vi "kursory.vi"() -> ()   [LabVIEW 2013]
uses:
  <vilib>/Utility/miscctls.llb/LVPointDoubleTypeDef.ctl
  <vilib>/Utility/miscctls.llb/LVCursorListTypeDef.ctl
  Kontrolki/GUI/Wysw_kursorow.ctl
  <vilib>/measure/NI_MABase.lvlib
panel:
  out "Data":T1
  in  "Create meas Cursor":bool
  in  "Delete cursor":bool
  in  "Create cursor":bool
  in  "Color Box":u32(colorbox)
  in  "Cursor List 2":T2
  in  "Free cursor":bool
  in  "stop":bool
  in  "Listbox":i32(listbox)
  out "Cursor List":T2
  out "Cursor.Cursor Position":T3
  out "Waveform Graph":waveform(dbl)[](graph)
  in  "Array":T4(array[cluster])=[{"signal type"=enum."Sine Wave", "frequency"=10.0, "amplitude"=2.0}, {"signal type"=enum."Sine Wave", "frequency"=13.0, "amplitude"=1.0}, {"signal type"=enum."Sine Wave", "frequency"=7.0, "amplitude"=1.0}, {"signal type"=enum."Sine Wave", "frequency"=5.0, "amplitude"=3.0}] {"amplitude" format="%0.2p"; "frequency" format="%0.2p"}
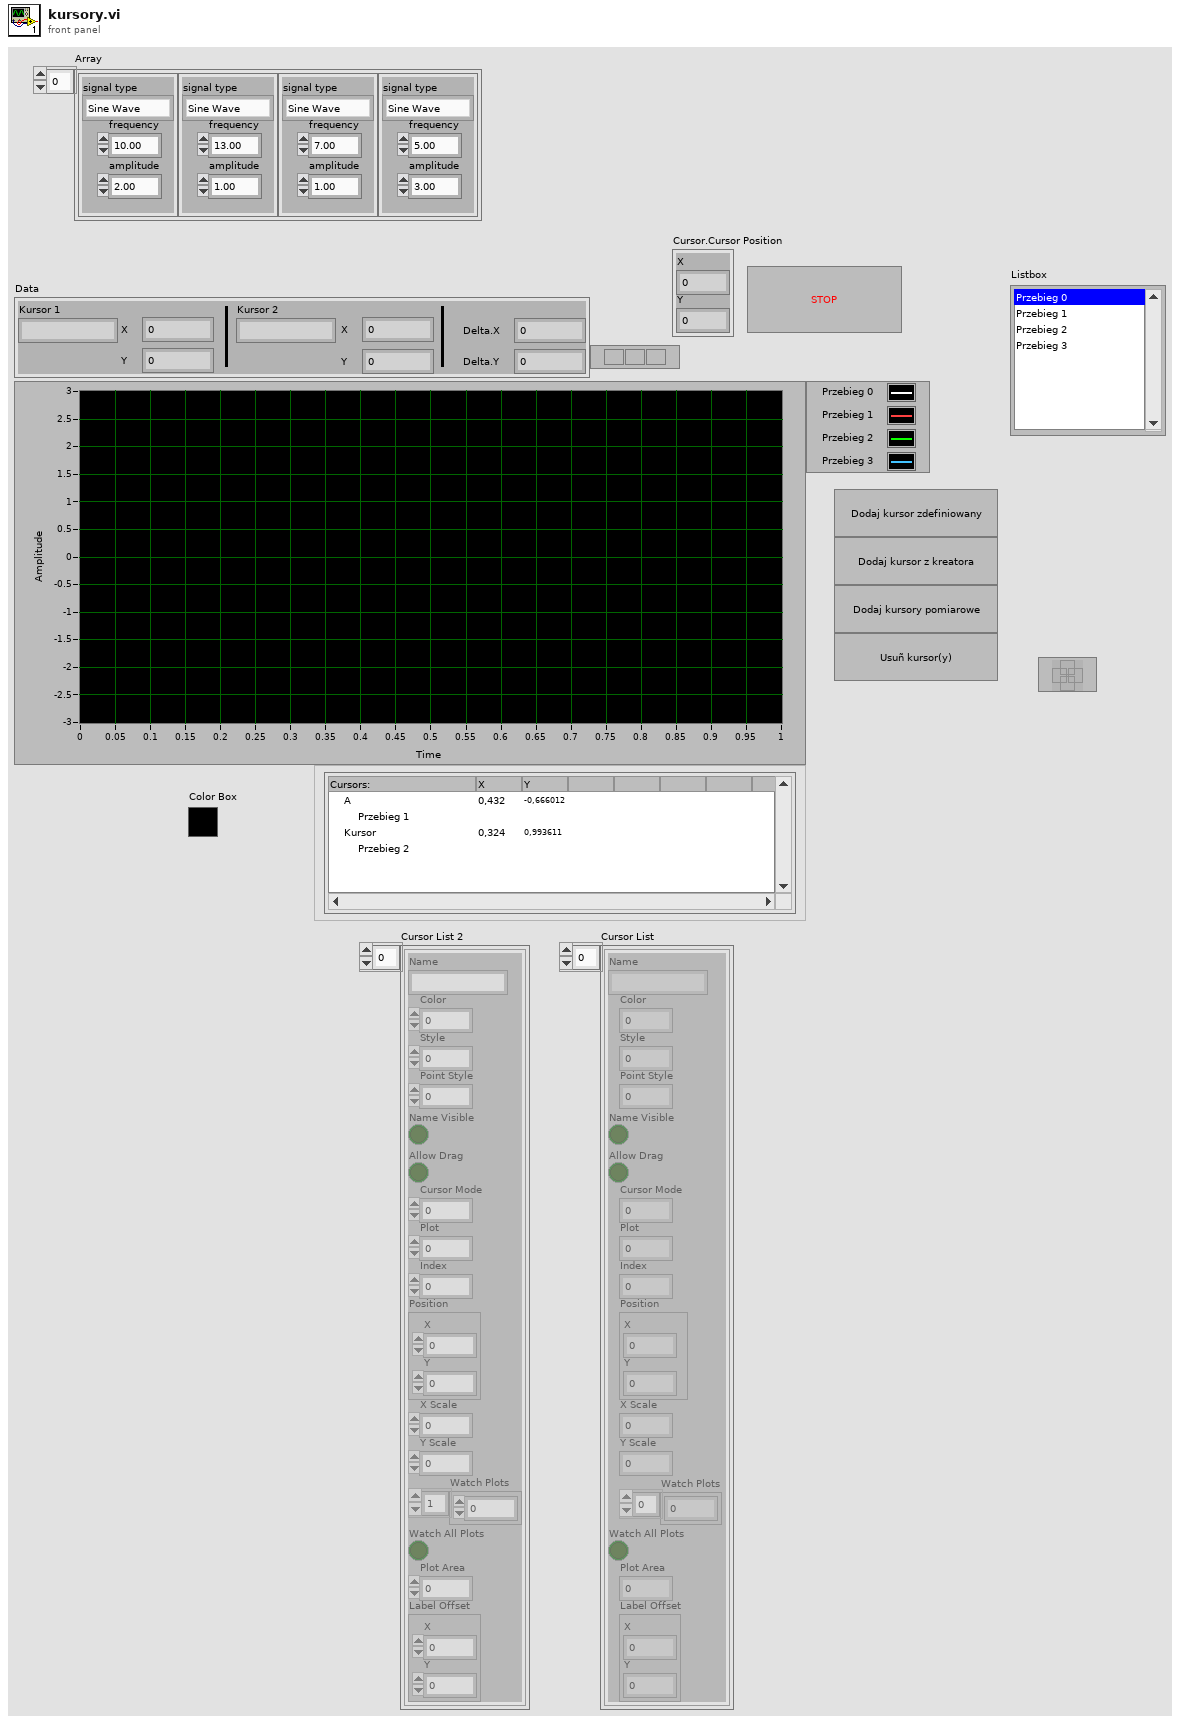
[diagram p1: front panel]
types:
  T1 = typedef "Wysw_kursorow.ctl" = cluster{"Pos.X1":dbl, "Pos.Y1":dbl, "Pos.X2":dbl, "Pos.Y2":dbl, "Delta.X":dbl, "Delta.Y":dbl, "Nazwa.1":string, "Nazwa.2":string}
  T2 = typedef "LVCursorListTypeDef.ctl" = cluster{"Name":string, "Color":u32, "Style":u8, "Point Style":u8, "Name Visible":bool, "Allow Drag":bool, "Cursor Mode":u32, "Plot":i32, "Index":i32, "Position":cluster{"X":dbl, "Y":dbl}, "X Scale":u32, "Y Scale":u32, "Watch Plots":i32[], "Watch All Plots":bool, "Plot Area":i32, "Label Offset":cluster{"X":dbl, "Y":dbl}}[]
  T3 = typedef "LVPointDoubleTypeDef.ctl" = cluster{"X":dbl, "Y":dbl}
  T4 = cluster{"signal type":enum16{"Sine Wave", "Triangle Wave", "Square Wave", "Sawtooth Wave"}, "frequency":dbl, "amplitude":dbl}[]
  T5 = enum16{"Sine Wave", "Triangle Wave", "Square Wave", "Sawtooth Wave"}
  T6 = cluster{"Name":string, "Color":u32, "Style":u8, "Point Style":u8, "Name Visible":bool, "Allow Drag":bool, "Cursor Mode":u32, "Plot":i32, "Index":i32, "Position":cluster{"X":dbl, "Y":dbl}, "X Scale":u32, "Y Scale":u32, "Watch Plots":i32[], "Watch All Plots":bool, "Plot Area":i32, "Label Offset":cluster{"X":dbl, "Y":dbl}}
  T7 = cluster{"Name":string, "Color":u32, "Style":u8, "Point Style":u8, "Name Visible":bool, "Allow Drag":bool, "Cursor Mode":u32, "Plot":i32, "Index":i32, "Position":cluster{"X":dbl, "Y":dbl}, "X Scale":u32, "Y Scale":u32, "Watch Plots":i32[], "Watch All Plots":bool, "Plot Area":i32, "Label Offset":cluster{"X":dbl, "Y":dbl}}[]
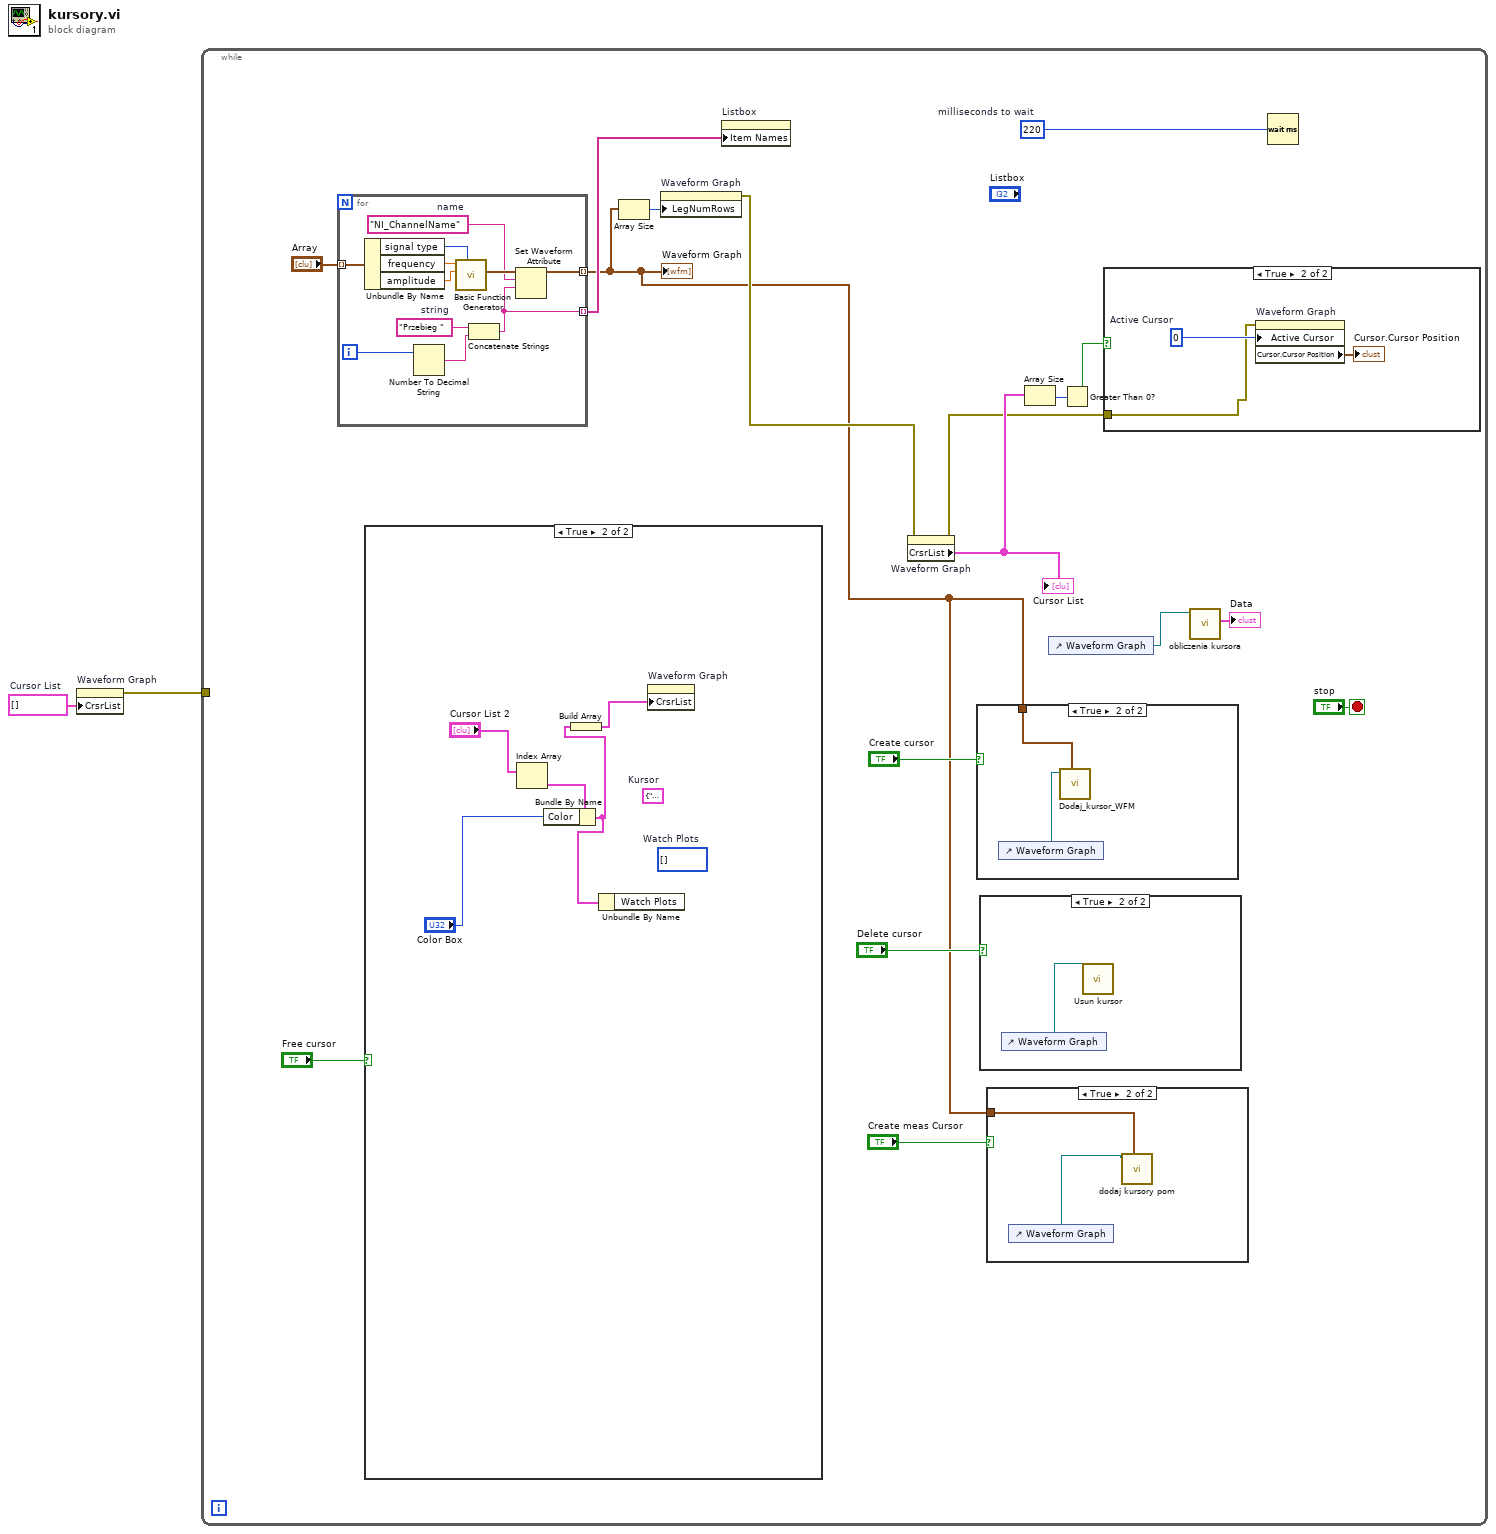
[diagram p0: block diagram]
diagram:
  w2 = T2 []  # Cursor List
  n1 = property on="Waveform Graph" class="WFGraph (strict)"("CrsrList"=w2) -> (error out=w1:errorcluster)  [unwired: 2 in, 1 out]
  n2 = while {
    tunnel: w1 -> [_]
    stop <- "stop" stop-if-true
    w15 = u32 220  # milliseconds to wait
    n3 = for {
      tunnel: "Array" -> [w40] mode=indexing
      tunnel: [w34] -> w4 mode=indexing
      tunnel: [w33] -> w17 mode=indexing
      i -> [w35]
      w37 = "Przebieg "  # string
      w38 = "NI_ChannelName"  # name
      n4 = Unbundle By Name(w40) -> ("signal type"=w43:T5, "frequency"=w42:dbl, "amplitude"=w41:dbl)
      n5 = Number To Decimal String(number=w35) -> (decimal integer string=w36:string)  [unwired: 1 in]
      n6 = call <vilib>:"Basic Function Generator.vi"("signal type"=w43, "amplitude"=w41, "frequency"=w42) -> ("signal out"=w39:waveform(dbl))  [unwired: 6 in, 2 out]
      n7 = Concatenate Strings(w37, w36) -> (w33:string)
      n8 = Set Waveform Attribute(5:w33, 6:w38, 7:w39) -> (3:w34:waveform(dbl))  [unwired: 1 in, 2 out]
    }
    "Waveform Graph" <- w4
    n9 = case shown="True" "Free cursor" {
      frame False {
      }
      frame True {
        (unwired) i32[] []  # Watch Plots
        (unwired) T6 {"Name"="", "Color"=0, "Style"=0, "Point Style"=0, "Name Visible"=FALSE, "Allow Drag"=FALSE, "Cursor Mode"=0, "Plot"=0, "Index"=0, "Position"={"X"=0.0, "Y"=0.0}, "X Scale"=0, "Y Scale"=0, "Watch Plots"=[], "Watch All Plots"=FALSE, "Plot Area"=0, "Label Offset"={"X"=0.0, "Y"=0.0}}  # Kursor
        n10 = Index Array(array="Cursor List 2") -> (element=w30:T6)  [unwired: 1 in]
        n11 = Bundle By Name(cluster=w30, "Color"="Color Box") -> (w28:T6)
        n12 = Build Array(w28) -> (w32:T7)
        n13 = Unbundle By Name(w28) -> ()  [unwired: 1 out]
        n14 = property on="Waveform Graph" class="WFGraph (strict)"("CrsrList"=w32) -> ()  [unwired: 2 in, 2 out]
      }
    }
    n15 = Array Size(array=w4) -> (size(s)=w18:i32)
    n16 = property on="Waveform Graph" class="WFGraph (strict)"("LegNumRows"=w18) -> (error out=w9:errorcluster)  [unwired: 2 in, 1 out]
    n17 = property on="Listbox" class="LstBox (strict)"("Item Names"=w17) -> ()  [unwired: 2 in, 2 out]
    n18 = property on="Waveform Graph" class="WFGraph (strict)"(error in=w9) -> (error out=w10:errorcluster, "CrsrList"=w13:T2)  [unwired: 1 in, 1 out]
    "Cursor List" <- w13
    n19 = case shown="True" "Create cursor" {
      tunnel: w4 -> [_ w24]
      frame False {
      }
      frame True {
        n20 = control-ref of="Waveform Graph"() -> (w23:refnum<vi>)
        n21 = call "Dodaj_kursor_WFM.vi"("Wektor przebiegow"=w24, "Wykres Ref"=w23) -> ()  [unwired: 9 in, 1 out]
      }
    }
    n22 = case shown="True" "Delete cursor" {
      frame False {
      }
      frame True {
        n23 = control-ref of="Waveform Graph"() -> (w22:refnum<vi>)
        n24 = call "Usun kursor.vi"("Wykres Ref"=w22) -> ()  [unwired: 10 in, 1 out]
      }
    }
    n25 = case shown="True" "Create meas Cursor" {
      tunnel: w4 -> [_ w20]
      frame False {
      }
      frame True {
        n26 = control-ref of="Waveform Graph"() -> (w21:refnum<vi>)
        n27 = call "dodaj kursory pom.vi"("Wektor przebiegow"=w20, "Wykres Ref"=w21) -> ()  [unwired: 9 in, 1 out]
      }
    }
    n28 = Array Size(array=w13) -> (size(s)=w12:i32)
    n29 = control-ref of="Waveform Graph"() -> (w7:refnum<vi>)
    n30 = Greater Than 0?(x=w12) -> (x > 0?=w11:bool)
    n31 = case shown="True" w11 {
      tunnel: w10 -> [_ w25]
      frame False {
      }
      frame True {
        w26 = u32 0  # Active Cursor
        n32 = property on="Waveform Graph" class="WFGraph (strict)"(error in=w25, "Active Cursor"=w26) -> ("Cursor.Cursor Position"=→"Cursor.Cursor Position":T3)  [unwired: 1 in, 2 out]
      }
    }
    n33 = call "obliczenia kursora.vi"("Wykres Ref"=w7) -> ("Data"=→"Data":T1)  [unwired: 9 in, 1 out]
    n34 = Wait (ms)(milliseconds to wait=w15) -> ()  [unwired: 1 out]
  }
